vi "PrintPaths.vi"(8 "error in (no error)":errorcluster, 11 "RunVITester in":refnum<class "RunVITester.lvclass">) -> (0 "error out":errorcluster, 3 "RunVITester out":refnum<class "RunVITester.lvclass">)   [LabVIEW 2027, in "RunVITester.lvclass"]
uses:
  RunVITester.lvclass
  <nishared>/LabVIEW CLI/Operations/CoreOperation/CoreOperation.lvclass/CoreOperation.ctl
  RunVITester.lvclass/RunVITester.ctl
  <nishared>/LabVIEW CLI/Operations/Utilities/Logger/Logger.lvclass
  <nishared>/LabVIEW CLI/Operations/CoreOperation/CoreOperation.lvclass
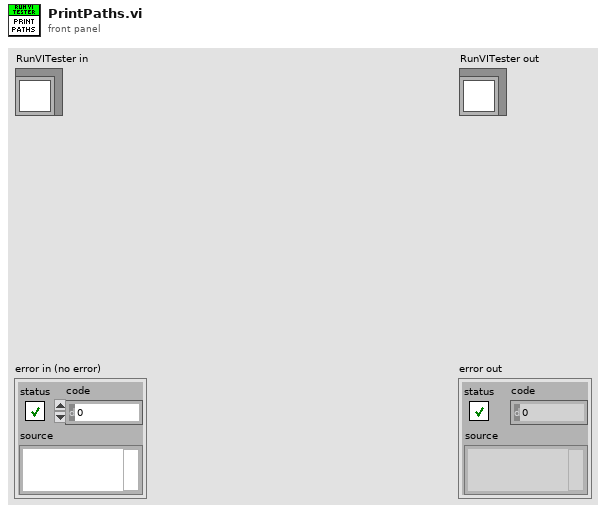
[diagram p1: front panel]
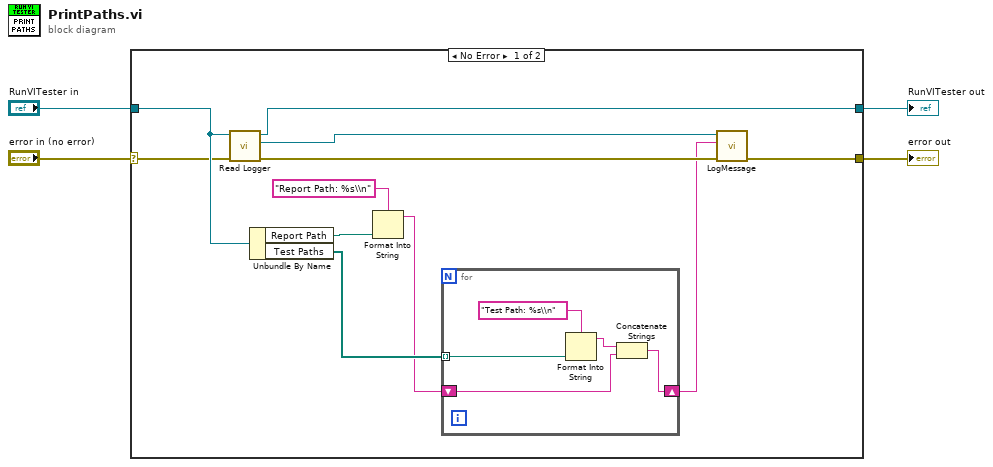
[diagram p0: block diagram]
diagram:
  n1 = case shown="No Error" "error in (no error)" {
    selector: "error in (no error)" -> [w9 w22]
    tunnel: [w8 w22] -> w3
    tunnel: [w15 w21] -> w1
    tunnel: "RunVITester in" -> [w12 w21]
    frame No Error {
      n2 = call <nishared>:"Read Logger.vi"("error in (no error)"=w9, "CoreOperation in"=w12) -> ("error out"=w13:errorcluster, "Logger.lvclass"=w14:refnum<class "Logger.lvclass">, "CoreOperation out"=w15:refnum<class "RunVITester.lvclass">)  [unwired: 7 in]
      n3 = Unbundle By Name(w12) -> ("Report Path"=w10:path, "Test Paths"=w7:path[])
      n4 = Format Into String(format string="Report Path: %s\\n", w10) -> (resulting string=w6:string)  [unwired: 2 in, 1 out]
      n5 = for {
        tunnel: w7 -> [w19] mode=indexing
        shift-right: [w16] -> w5
        shift-left: w6 -> [w17]
        n6 = Format Into String(format string="Test Path: %s\\n", w19) -> (resulting string=w18:string)  [unwired: 2 in, 1 out]
        n7 = Concatenate Strings(w18, w17) -> (w16:string)
      }
      n8 = call <nishared>:"LogMessage.vi"("error in (no error)"=w13, "Message"=w5, "Logger in"=w14) -> ("error out"=w8:errorcluster)  [unwired: 7 in, 1 out]
    }
    frame Error {
    }
  }
  "error out" <- w3
  "RunVITester out" <- w1
